vi "Abreviate Name.vi"(10 "Max Length":i32, 11 "Long Name in":string) -> (3 "Long Name out":string)   [LabVIEW 2020, in "Pure Mock Class Generator.lvclass"]
uses:
  Pure Mock Class Generator.lvclass
  Pure Mock Class Generator.lvclass/Pure Mock Class Generator.ctl
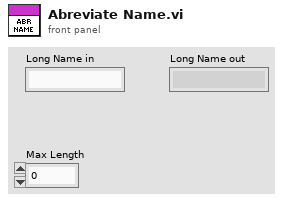
[diagram p1: front panel]
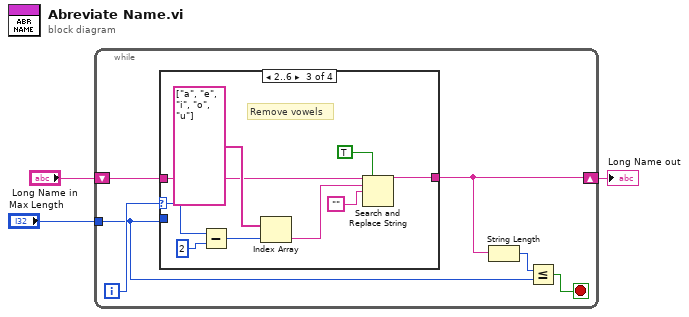
[diagram p0: block diagram]
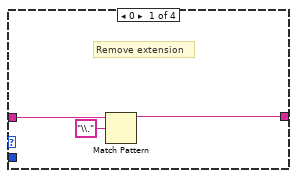
[diagram p2: hidden frame]
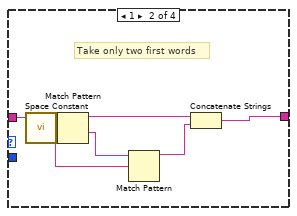
[diagram p3: hidden frame]
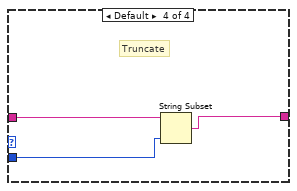
[diagram p4: hidden frame]
diagram:
  n1 = while {
    shift-right: [w5] -> w2
    shift-left: "Long Name in" -> [w8]
    tunnel: "Max Length" -> [w4]
    i -> [w9]
    stop <- w6 stop-if-true
    n2 = case shown="2..6" w9 {
      selector: w9 -> [_ _ w26 _]
      tunnel: w8 -> [w12 w18 w23 w30]
      tunnel: [w10 w15 w22 w29] -> w5
      tunnel: w4 -> [_ _ _ w28]
      frame 0 {
        # "Remove extension"
        n3 = Match Pattern(string=w12, regular expression="\\.") -> (before substring=w10:string)  [unwired: 1 in, 3 out]
      }
      frame 1 {
        # "Take only two first words"
        n4 = call <vilib>:"Space Constant.vi"() -> ("String"=w16:string)
        n5 = Match Pattern(string=w18, regular expression=w16) -> (before substring=w17:string, after substring=w13:string)  [unwired: 1 in, 2 out]
        n6 = Match Pattern(string=w13, regular expression=w16) -> (before substring=w14:string)  [unwired: 1 in, 3 out]
        n7 = Concatenate Strings(w17, w14) -> (w15:string)
      }
      frame 2..6 {
        # "Remove vowels"
        n8 = Subtract(x=w26, y=2) -> (x-y=w25:i32)
        n9 = Index Array(array=string[] ["a", "e", "i", "o", "u"], index=w25) -> (element=w20:string)
        n10 = Search and Replace String(replace all?=TRUE ("replace all? (F)"), input string=w23, search string=w20, replace string="") -> (result string=w22:string)  [unwired: 4 in, 3 out]
      }
      frame Default {
        # "Truncate"
        n11 = String Subset(string=w30, length (rest)=w28) -> (substring=w29:string)  [unwired: 1 in]
      }
    }
    n12 = String Length(string=w5) -> (length=w7:i32)
    n13 = Less Or Equal?(x=w7, y=w4) -> (x <= y?=w6:bool)
  }
  "Long Name out" <- w2
